vi "request file path.vi"(8 "error in (no error)":errorcluster, 11 "Data Log in":refnum<class "Data Log.lvclass">=refnum) -> (0 "error out":errorcluster, 2 "csv File Path":path caption="selected path", 3 "Data Log out":refnum<class "Data Log.lvclass">)   [LabVIEW 2025, in "Data Log.lvlib" / "generic data log.lvclass"]
uses:
  generic data log.lvclass
  generic data log.lvclass/generic data log.ctl
  <vilib>/Utility/sysdir.llb/System Directory Type.ctl
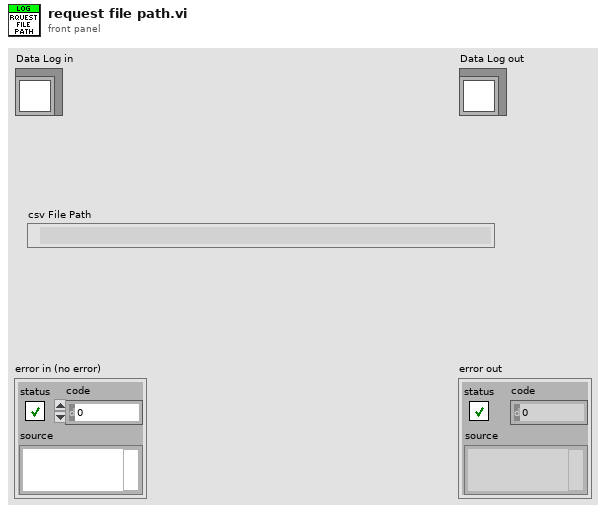
[diagram p1: front panel]
types:
  T1 = typedef "System Directory Type.ctl" = i32
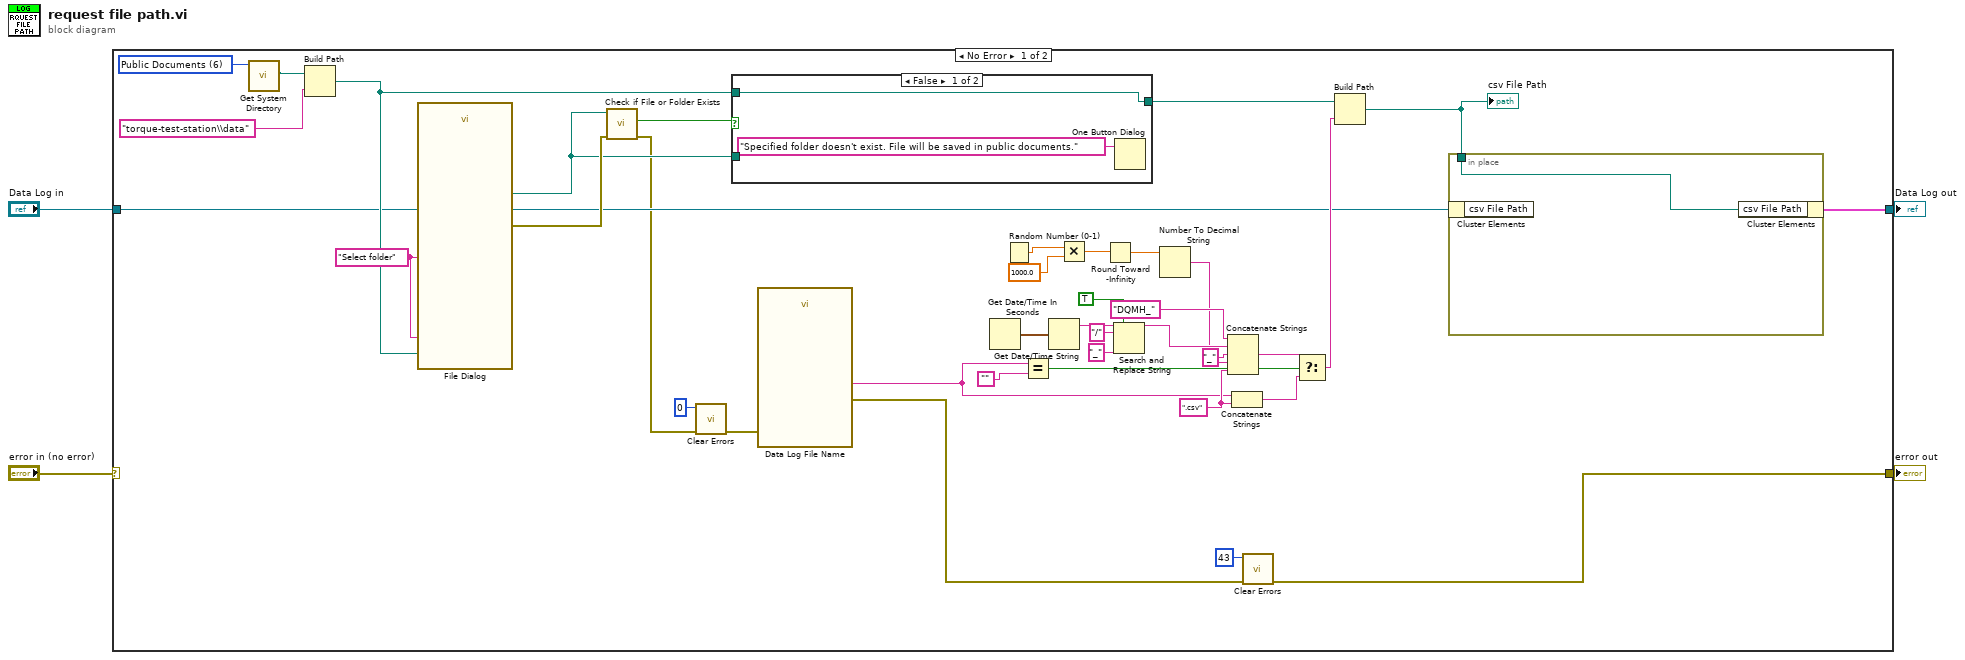
[diagram p0: block diagram]
diagram:
  n1 = case shown="No Error" "error in (no error)" {
    selector: "error in (no error)" -> [_ w48]
    tunnel: [w8 w48] -> w3
    tunnel: [w10 w47] -> w1
    tunnel: "Data Log in" -> [w11 w47]
    frame No Error {
      w22 = ".csv" ("string")
      w17 = "Select folder" ("button label")
      w12 = T1 6 items=["User Home"=0, "User Desktop"=1, "User Documents"=2, "User Application Data"=3, "User Preferences"=4, "User Temporary"=5, "Public Documents"=6, "Public Application Data"=7, "Public Preferences"=8, "Public Cache"=13, "System Core Libraries"=9, "System Installed Libraries"=10, "Application Files"=11, "Boot Volume Root"=12] ("system directory type")
      n2 = call <vilib>:"Get System Directory.vi"("system directory type"=w12) -> ("system directory"=w42:path)  [unwired: 10 in]
      n3 = Build Path(base path=w42, name or relative path="torque-test-station\\data") -> (appended path=w13:path)
      n4 = call "File Dialog"("start path"=w13, "prompt"=w17, "button label"=w17) -> ("selected path"=w14:path, "error out"=w24:errorcluster)  [unwired: 9 in, 2 out]
      n5 = call <vilib>:"Check if File or Folder Exists.vi"("error in (no error)"=w24, "path"=w14) -> ("error out"=w7:errorcluster, "file or folder exists?"=w16:bool)  [unwired: 7 in, 1 out]
      n6 = call <vilib>:"Clear Errors.vi"("error in (no error)"=w7, "specific error code to clear (0: all)"=0) -> ("error out"=w6:errorcluster)  [unwired: 4 in, 1 out]
      n7 = case shown="False" w16 {
        tunnel: [w45 w46] -> w15
        tunnel: w14 -> [_ w46]
        tunnel: w13 -> [w45 _]
        frame False {
          n8 = One Button Dialog(message="Specified folder doesn't exist. File will be saved in public documents.") -> ()  [unwired: 1 in, 1 out]
        }
        frame True {
        }
      }
      n9 = call "Data Log File Name"("error in (no error)"=w6) -> ("File name"=w21:string, "error out"=w18:errorcluster)  [unwired: 16 in, 1 out]
      n10 = Get Date/Time In Seconds() -> (seconds since 1Jan1904=w38:timestamp)
      n11 = Random Number (0-1)() -> (number: 0 to 1=w30:dbl)
      n12 = Equal?(x=w21, y="") -> (x = y?=w39:bool)
      n13 = Get Date/Time String(seconds (now)=w38) -> (date string=w37:string)  [unwired: 2 in, 1 out]
      n14 = Multiply(x=w30, y=1000.0) -> (x*y=w28:dbl)
      n15 = Round Toward -Infinity(1:w28) -> (0:w27:dbl)
      n16 = Search and Replace String(replace all?=TRUE ("replace all? (F)"), input string=w37, search string="/", replace string="_" ("replace string (\"\")")) -> (result string=w34:string)  [unwired: 4 in, 3 out]
      n17 = Number To Decimal String(number=w27) -> (decimal integer string=w26:string)  [unwired: 1 in]
      n18 = Concatenate Strings("DQMH_" ("string"), w34, "_" ("string"), w26, w22) -> (w32:string)
      n19 = Concatenate Strings(w21, w22) -> (w20:string)
      n20 = call <vilib>:"Clear Errors.vi"("error in (no error)"=w18, "specific error code to clear (0: all)"=43) -> ("error out"=w8:errorcluster)  [unwired: 4 in, 1 out]
      n21 = Select(t=w32, s=w39, f=w20) -> (s? t:f=w23:string)
      n22 = Build Path(base path=w15, name or relative path=w23) -> (appended path=w9:path)
      "csv File Path" <- w9
      n23 = in-place {
        in-place-border: w9 -> [w43]
        n24 = in-place-cluster #1(w11) -> ()  [unwired: 1 out]
        n25 = in-place-cluster #1("csv File Path"=w43) -> (w10:cluster{})
      }
    }
    frame Error {
    }
  }
  "error out" <- w3
  "Data Log out" <- w1
